vi "Step UI Main.vi"(8 "error in (no error)":errorcluster, 10 "Parameters":T1, 11 "Wait Step UI in":refnum<class "Wait Step UI.lvclass">) -> (0 "error out":errorcluster, 3 "Wait Step UI out":refnum<class "Wait Step UI.lvclass">)   [LabVIEW 2015, in "Wait Step UI.lvclass"]
uses:
  Wait Step UI.lvclass
  classes/Step/UI/Controls/Step UI Main Parameters.ctl
  <vilib>/NI/AMC/Message Queue.ctl
  <vilib>/NI/AMC/Message.ctl
  <vilib>/NI/Tools/Keyed Array/KeyedArray.ctl
  Editor/Classes/StepNode/StepNode.lvclass
  <vilib>/NI/Configuration Framework/Node/UserEventRef.ctl
  <vilib>/NI/Configuration Framework/Controls/EventCluster.ctl
  Config/Wait Step Config.lvclass
  <vilib>/NI/AMC/Create Single Message.vi
  <vilib>/NI/AMC/Update Message Routing Info.vi
  <vilib>/NI/AMC/Send Message.vi
  <vilib>/NI/AMC/AMC.lvlib
  <vilib>/NI/Configuration Framework/Node/NISE_CEF_Node.lvclass
  <vilib>/NI/Configuration Framework/NISE_CEF_TreeControl.lvlib
  <vilib>/NI/Tools/Keyed Array/Tools_KeyedArray.lvlib
  classes/Step/UI/Step UI.lvclass
panel:
  in  "Wait (ms)":u32
  out "current time":timestamp
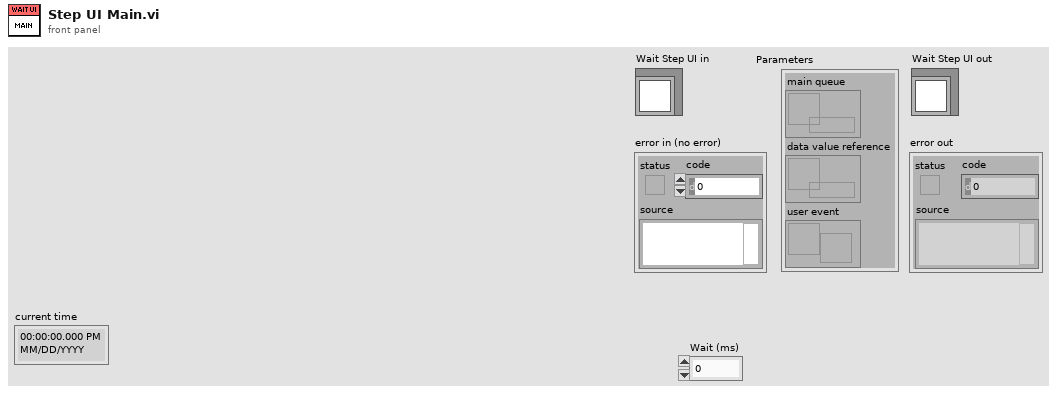
[diagram p1: front panel]
types:
  T1 = typedef "Step UI.lvclass/Step UI Main Parameters.ctl" = cluster{"main queue":T2, "data value reference":refnum<data-value>, "user event":T3}
  T2 = typedef "AMC.lvlib/Message Queue.ctl" = refnum<queue>
  T3 = typedef "NISE_CEF_Node.lvclass/UserEventRef.ctl" = refnum<user-event>
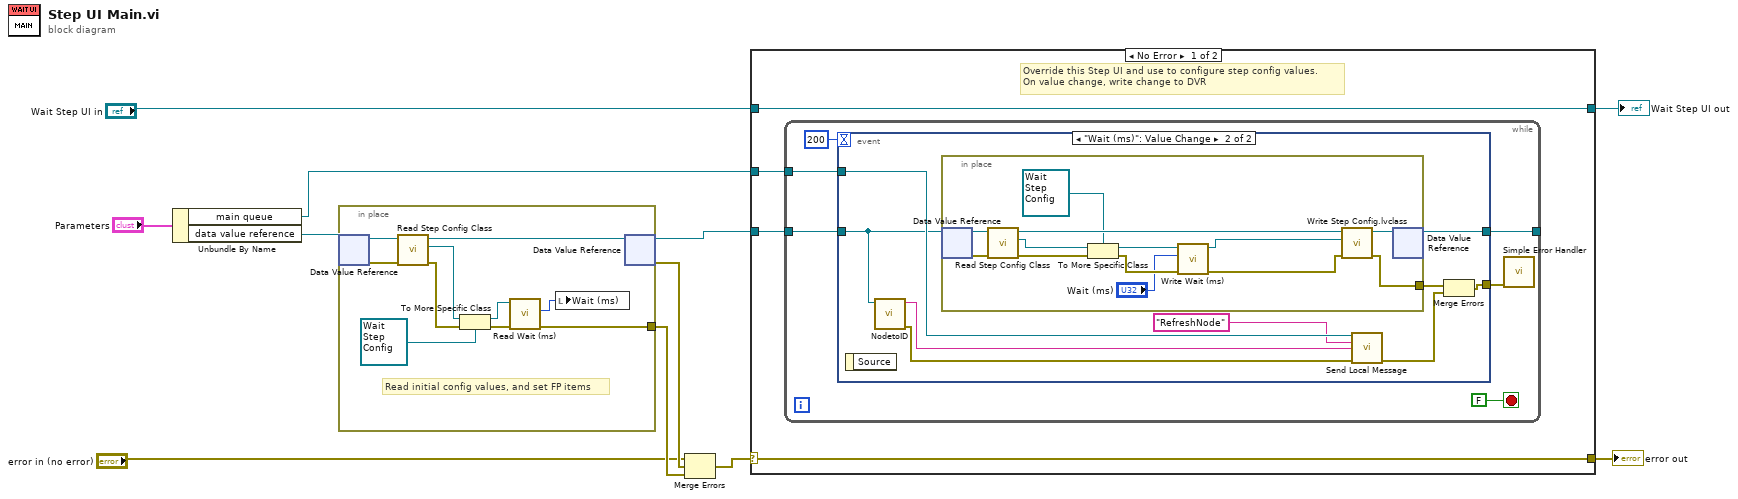
[diagram p0: block diagram]
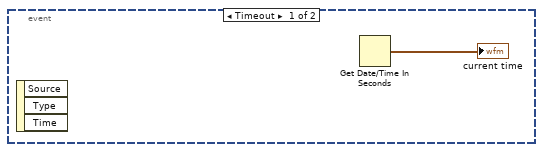
[diagram p2: hidden frame]
diagram:
  n1 = Unbundle By Name("Parameters") -> ("main queue"=w6:T2, "data value reference"=w7:refnum<data-value>)
  n2 = in-place "In Place Element Structure" {
    in-place-border: [w18] -> w8
    # "Read initial config values, and set FP items"
    n3 = in-place-dvr #1(w7) -> (w21:refnum<class "StepNode.lvclass">, w19:errorcluster)
    n4 = call-dynamic "Read Step Config Class.vi"("error in (no error)"=w19, "StepNode in"=w21) -> ("error out"=w17:errorcluster, "Step Config.lvclass"=w13:refnum<class "Step Config.lvclass">, "StepNode out"=w20:refnum<class "StepNode.lvclass">)  [unwired: 7 in]
    n5 = To More Specific Class(target class=refnum<class "Wait Step Config.lvclass"> refnum ("Wait Step Config.lvclass"), reference=w13, error in=w17) -> (specific class reference=w14:refnum<class "Wait Step Config.lvclass">, error out=w16:errorcluster)
    n6 = call-dynamic "Read Wait (ms).vi"("error in (no error)"=w16, "Wait Step in"=w14) -> ("error out"=w18:errorcluster, "Wait (ms)"=w12:u32)  [unwired: 7 in, 1 out]
    n7 = local write "Wait (ms)"(w12) -> ()
    n8 = in-place-dvr #1(w20) -> (w11:refnum<data-value>, w9:errorcluster)
  }
  n9 = Merge Errors("error in (no error)", w9, w8) -> (w10:errorcluster)
  n10 = case shown="No Error" w10 {
    selector: w10 -> [w24 w56]
    tunnel: [w24 w56] -> w4
    tunnel: [w25 w55] -> w5
    tunnel: "Wait Step UI in" -> [w25 w55]
    tunnel: w11 -> [w23 _]
    tunnel: w6 -> [w22 _]
    frame No Error {
      # "Override this Step UI and use to configure step config values.\nOn value change, write change to DVR"
      n11 = while {
        tunnel: w23 -> [w29]
        tunnel: [w28] -> _
        tunnel: w22 -> [w26]
        stop <- FALSE stop-if-true
        n12 = event shown="[1] \"Wait (ms)\": Value Change" {
          selector: _ -> [_ _]
          dyn-events: _ -> [_ _]
          timeout: 200 -> [_ _]
          tunnel: w29 -> [_ w35]
          tunnel: [_ w41] -> w28
          tunnel: [_ w38] -> w27
          tunnel: w26 -> [_ w39]
          event Timeout {
            n13 = event-data() -> ()  [unwired: 1 in, 3 out]
            n14 = Get Date/Time In Seconds() -> (seconds since 1Jan1904=→"current time":timestamp)
          }
          event "Wait (ms)": Value Change {
            n15 = event-data() -> ()  [unwired: 1 in, 1 out]
            n16 = call <vilib>:"NodetoID.vi"("node ref"=w35) -> ("error out"=w33:errorcluster, "ID"=w34:string)  [unwired: 9 in]
            n17 = in-place {
              in-place-border: [w50] -> w40
              n18 = in-place-dvr #2(w35) -> (w54:refnum<class "StepNode.lvclass">, w53:errorcluster)
              n19 = call-dynamic "Read Step Config Class.vi"("error in (no error)"=w53, "StepNode in"=w54) -> ("error out"=w44:errorcluster, "Step Config.lvclass"=w46:refnum<class "Step Config.lvclass">, "StepNode out"=w52:refnum<class "StepNode.lvclass">)  [unwired: 7 in]
              n20 = To More Specific Class(target class=refnum<class "Wait Step Config.lvclass"> refnum ("Wait Step Config.lvclass"), reference=w46, error in=w44) -> (specific class reference=w47:refnum<class "Wait Step Config.lvclass">, error out=w43:errorcluster)
              n21 = call-dynamic "Write Wait (ms).vi"("error in (no error)"=w43, "Wait (ms)"="Wait (ms)", "Wait Step in"=w47) -> ("error out"=w49:errorcluster, "Wait Step out"=w48:refnum<class "Wait Step Config.lvclass">)  [unwired: 7 in]
              n22 = call-dynamic "Write Step Config.lvclass.vi"("error in (no error)"=w49, "Step Config.lvclass"=w48, "StepNode in"=w52) -> ("error out"=w50:errorcluster, "StepNode out"=w51:refnum<class "StepNode.lvclass">)  [unwired: 7 in]
              n23 = in-place-dvr #2(w51) -> (w41:refnum<data-value>)  [unwired: 1 out]
            }
            n24 = call <vilib>:"Send Local Message.vi"("message queue in"=w39, "message name"="RefreshNode", "message value"=w34, "error in"=w33) -> ("error out"=w37:errorcluster)  [unwired: 9 in, 2 out]
            n25 = Merge Errors(w40, w37) -> (w38:errorcluster)
          }
        }
        n26 = call <vilib>:"Simple Error Handler.vi"("error in (no error)"=w27) -> ()  [unwired: 4 in, 5 out]
      }
    }
    frame Error {
    }
  }
  "error out" <- w4
  "Wait Step UI out" <- w5
